vi "Main_Motor_old.vi"(0 "VISA resource name":refnum<visa-resource-name>, 1 "Old Position Motor":dbl, 2 "Old Current load":dbl, 5 "Motor ID":u8, 7 "Address":u8=14, 9 "Torque enable?":bool, 11 "error in (no error)":errorcluster, 12 "Goal Position":dbl=150.0, 13 "Goal Speed (RPM)":dbl) -> (4 "VISA resource name out":refnum<visa-resource-name>, 6 "New Position Motor":dbl, 8 "New Current load (mA)":dbl, 15 "error out":errorcluster)   [LabVIEW 2015]
uses:
  <instrlib>/Dynamixel Motor/Dynamixel Motor.lvlib
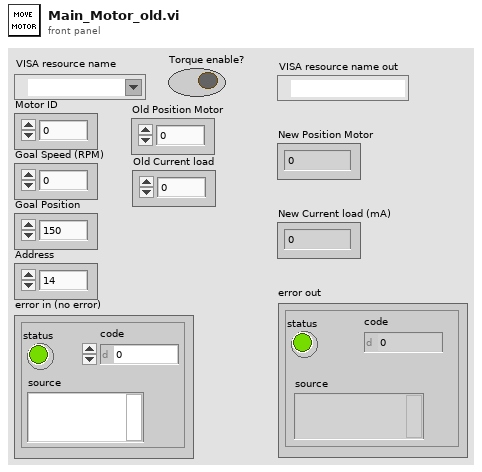
[diagram p1: front panel]
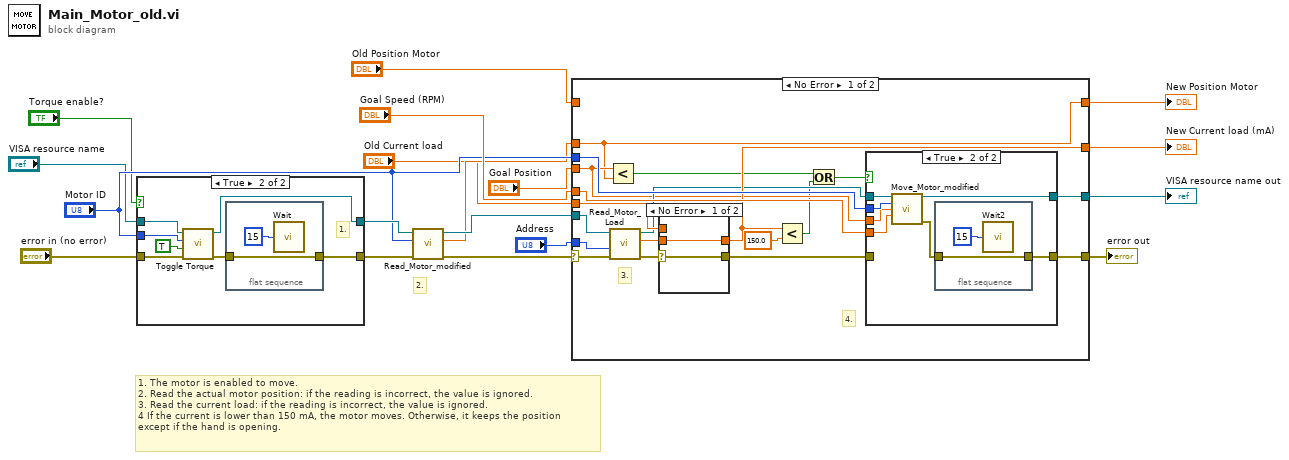
[diagram p0: block diagram]
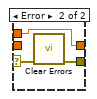
[diagram p3: hidden frame]
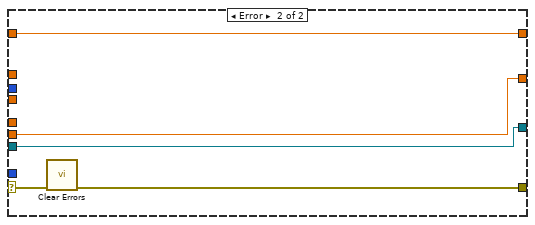
[diagram p4: hidden frame]
diagram:
  # "2."
  # "1. The motor is enabled to move.\n2. Read the actual motor position: if the reading is incorrect, the value is ignored.\n3. Read the current load: if the reading is incorrect, the value is ignored.\n4 If the current is lower than 150 mA, the motor moves. Otherwise, it keeps the position \nexcept if the hand is opening."
  n1 = case shown="True" "Torque enable?" {
    tunnel: "VISA resource name" -> [w20 w27]
    tunnel: [w20 w26] -> w16
    tunnel: "error in (no error)" -> [w19 w25]
    tunnel: [w19 w21] -> w17
    tunnel: "Motor ID" -> [_ w24]
    frame False {
    }
    frame True {
      # "1."
      n2 = call <instrlib>:"Toggle Torque.vi"("error in (no error)"=w25, "Toggle torque (OFF)"=TRUE, "Motor ID (0)"=w24, "VISA resource name"=w27) -> ("error out"=w22:errorcluster, "VISA resource name out"=w26:refnum<visa-resource-name>)  [unwired: 6 in]
      n3 = flat-sequence {
        tunnel: w22 -> [w28]
        tunnel: [w28] -> w21
        frame #0 {
          n4 = call "Wait"("Count(mSec)"=u32 15) -> ()  [unwired: 1 out]
        }
      }
    }
  }
  n5 = call "Read_Motor_modified.vi"("error in (no error)"=w17, "Motor ID (0)"="Motor ID", "VISA Refnum in"=w16) -> ("error out"=w4:errorcluster, "Position"=w8:dbl, "VISA Refnum out"=w15:refnum<visa-resource-name>)  [unwired: 6 in]
  n6 = case shown="No Error" w4 {
    selector: w4 -> [w44 w67]
    tunnel: "Goal Speed (RPM)" -> [w48 _]
    tunnel: [w36 w68] -> w6
    tunnel: w15 -> [w45 w68]
    tunnel: "Motor ID" -> [w47 _]
    tunnel: "Goal Position" -> [w35 _]
    tunnel: [w34 w69] -> w9
    tunnel: w8 -> [w34 _]
    tunnel: "Address" -> [w43 _]
    tunnel: [w46 w66] -> w7
    tunnel: "Old Position Motor" -> [_ w69]
    tunnel: [w40 w65] -> w2
    tunnel: "Old Current load" -> [w41 w65]
    frame No Error {
      # "4."
      # "3."
      n7 = Less?(x=w35, y=w34) -> (x < y?=w33:bool)
      n8 = call "Read_Motor_Load.vi"("error in (no error)"=w44, "Address"=w43, "VISA Refnum in"=w45) -> ("error out"=w38:errorcluster, "Current load"=w42:dbl, "VISA Refnum out"=w37:refnum<visa-resource-name>)  [unwired: 6 in]
      n9 = case shown="No Error" w38 {
        selector: w38 -> [w60 w63]
        tunnel: [w61 w64] -> w40
        tunnel: w42 -> [w61 _]
        tunnel: w41 -> [_ w64]
        tunnel: [w60 w62] -> w30
        frame No Error {
        }
        frame Error {
          n10 = call <vilib>:"Clear Errors.vi"("error in (no error)"=w63) -> ("error out"=w62:errorcluster)  [unwired: 5 in, 1 out]
        }
      }
      n11 = Less?(x=w40, y=150.0) -> (x < y?=w32:bool)
      n12 = Or(x=w33, y=w32) -> (x .or. y?=w31:bool)
      n13 = case shown="True" w31 {
        tunnel: w48 -> [_ w57]
        tunnel: w47 -> [_ w56]
        tunnel: w35 -> [_ w55]
        tunnel: [w49 w53] -> w46
        tunnel: w37 -> [w50 w52]
        tunnel: [w50 w51] -> w36
        tunnel: w30 -> [w49 _]
        frame False {
        }
        frame True {
          n14 = call "Move_Motor_modified.vi"("VISA Refnum in"=w52, "Motor ID (0)"=w56, "Goal Position (bit)"=w55, "Goal Speed (RPM)"=w57) -> ("VISA Refnum out"=w51:refnum<visa-resource-name>, "error out"=w54:errorcluster)  [unwired: 10 in]
          n15 = flat-sequence {
            tunnel: w54 -> [w58]
            tunnel: [w58] -> w53
            frame #0 {
              n16 = call "Wait2"("Count(mSec)"=u32 15) -> ()  [unwired: 1 out]
            }
          }
        }
      }
    }
    frame Error {
      n17 = call <vilib>:"Clear Errors.vi"("error in (no error)"=w67) -> ("error out"=w66:errorcluster)  [unwired: 5 in, 1 out]
    }
  }
  "VISA resource name out" <- w6
  "New Position Motor" <- w9
  "error out" <- w7
  "New Current load (mA)" <- w2
